vi "Jitter Benchmark (Win).vi"() -> ()   [LabVIEW 2013]
doc: "This example uses an assembly-level call to obtain precise timestamps from RT targets. The purpose of this example is to gather timing information on a user's VI by running it for several iterations. The example obtains several consecutive 64-bit timestamps, which are stored in an array and used later to produce a histogram of execution time. This VI can self-calibrate by subtracting out the overhead of calling NI Get Timestamp.vi from the array of timing data.\n\nINSTRUCTIONS:\n1. Select a number of iterations and warmup iterations to exclude from the benchmark.\n2. Use calibration if you want to exclude the overhead of the timestamping operation.\n3. Go to the diagram and insert the code you want to benchmark."
uses:
  Support/_RTUtility_win.llb/NI Timestamp.ctl
panel:
  in  "Tab Control":enum32{"Results", "Configure"}(tab)
  in  "Target Period":u32=2 caption="msec"
  out "Max jitter":dbl caption="usec" format="%.2f"
  out "Average period":dbl caption="usec" format="%.2f"
  in  "Calibrate?":bool
  in  "Warmup iterations":i32=10
  in  "Iterations":i32=500
  in  "stop":bool
  out "Execution Times":dbl[](graph)
  # "Windows Jitter Benchmark"
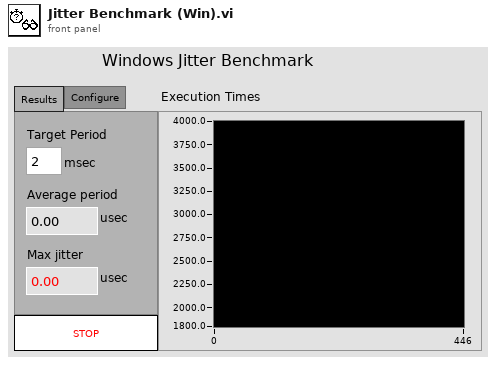
[diagram p1: front panel]
types:
  T1 = typedef "NI Timestamp.ctl" = cluster{"H32":u32, "L32":u32}
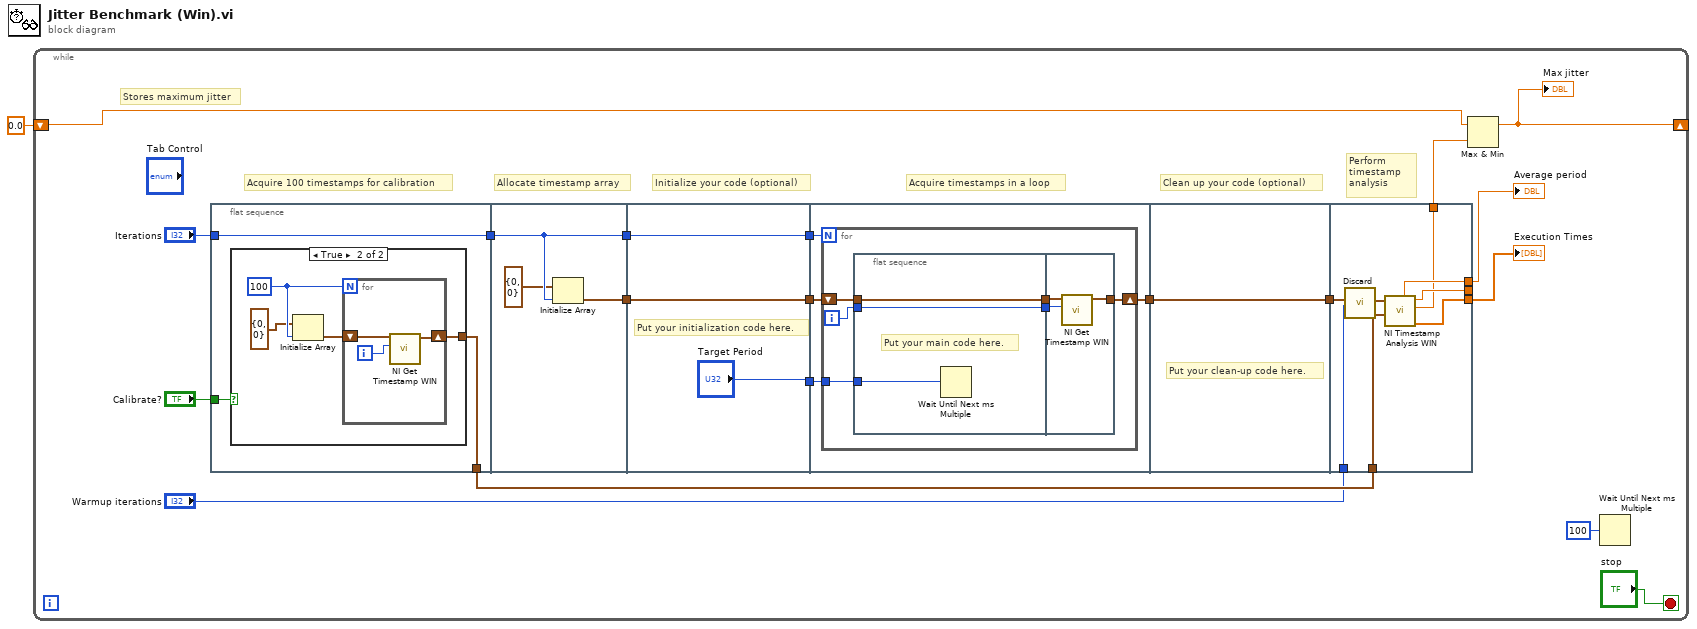
[diagram p0: block diagram]
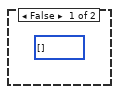
[diagram p2: hidden frame]
diagram:
  n1 = while {
    shift-right: [w4] -> _
    shift-left: 0.0 -> [w2]
    stop <- "stop" stop-if-true
    # "Stores maximum jitter"
    # "Perform timestamp analysis"
    # "Acquire timestamps in a loop"
    # "Clean up your code (optional)"
    # "Initialize your code (optional)"
    # "Allocate timestamp array"
    # "Acquire 100 timestamps for calibration"
    n2 = flat-sequence {
      tunnel: "Iterations" -> [w23]
      tunnel: [w23] -> w20
      tunnel: "Calibrate?" -> [w22]
      tunnel: [w21] -> w10
      tunnel: [w32] -> w19
      tunnel: [w33] -> w18
      tunnel: w20 -> [w32]
      tunnel: [w36] -> w17
      tunnel: [w35] -> w16
      tunnel: w19 -> [w36]
      tunnel: w18 -> [w35]
      tunnel: ["Target Period"] -> w15
      tunnel: [w40] -> w14
      tunnel: w17 -> [w39]
      tunnel: w16 -> [w38]
      tunnel: w15 -> [w37]
      tunnel: w14 -> [w53]
      tunnel: [w53] -> w13
      tunnel: w13 -> [w55]
      tunnel: w10 -> [w57]
      tunnel: [w59] -> w3
      tunnel: [w60] -> _
      tunnel: [w58] -> w9
      tunnel: "Warmup iterations" -> [w54]
      tunnel: [w61] -> w7
      frame #0 {
        n3 = case shown="True" w22 {
          tunnel: [_ w27] -> w21
          frame False {
            (unwired) u64[] []
          }
          frame True {
            w25 = 100
            n4 = Initialize Array(T1 {"H32"=0, "L32"=0} ("Timestamp"), w25) -> (w26:T1[])
            n5 = for {
              N: w25 -> [_]
              shift-right: [w29] -> w27
              shift-left: w26 -> [w28]
              i -> [w30]
              n6 = call "NI Get Timestamp WIN.vi"("iteration"=w30, "timestamp array in"=w28) -> ("timestamp array in out"=w29:T1[])  [unwired: 1 in, 8 out]
            }
          }
        }
      }
      frame #1 {
        n7 = Initialize Array(T1 {"H32"=0, "L32"=0} ("Timestamp"), w32) -> (w33:T1[])
      }
      frame #2 {
        # "Put your initialization code here."
      }
      frame #3 {
        n8 = for {
          N: w39 -> [_]
          shift-right: [w46] -> w40
          shift-left: w38 -> [w45]
          tunnel: w37 -> [w41]
          i -> [w44]
          n9 = flat-sequence {
            tunnel: w45 -> [w49]
            tunnel: [w49] -> w43
            tunnel: w44 -> [w48]
            tunnel: [w48] -> w42
            tunnel: w41 -> [w47]
            tunnel: [w52] -> w46
            tunnel: w43 -> [w51]
            tunnel: w42 -> [w50]
            frame #0 {
              # "Put your main code here."
              n10 = Wait Until Next ms Multiple(millisecond multiple=w47) -> ()  [unwired: 1 out]
            }
            frame #1 {
              n11 = call "NI Get Timestamp WIN.vi"("iteration"=w50, "timestamp array in"=w51) -> ("timestamp array in out"=w52:T1[])  [unwired: 1 in, 8 out]
            }
          }
        }
      }
      frame #4 {
        # "Put your clean-up code here."
      }
      frame #5 {
        n12 = call "Discard.vi"("count array"=w55, "% to discard"=w54) -> ("Array out"=w56:T1[])  [unwired: 17 out]
        n13 = call "NI Timestamp Analysis WIN.vi"("calibration array in"=w57, "timestamp array in"=w56) -> ("loop execution time (uS)"=w58:dbl[], "max jitter (uS)"=w59:dbl, "std dev (uS)"=w60:dbl, "mean (uS)"=w61:dbl)  [unwired: 1 in, 5 out]
      }
    }
    n14 = Max & Min(x=w2, y=w3) -> (max(x,y)=w4:dbl)  [unwired: 1 out]
    "Max jitter" <- w4
    n15 = Wait Until Next ms Multiple(millisecond multiple=u32 100) -> ()  [unwired: 1 out]
    "Execution Times" <- w9
    "Average period" <- w7
  }
